vi "Read id.vi"(8 "error in (no error)":errorcluster, 11 "IDable in":refnum<class "IDable.lvclass">) -> (0 "error out":errorcluster, 2 "id":string, 3 "IDable out":refnum<class "IDable.lvclass">)   [LabVIEW 2017, in "IDable.lvclass"]
uses:
  IDable.lvclass
  IDable.lvclass/IDable.ctl
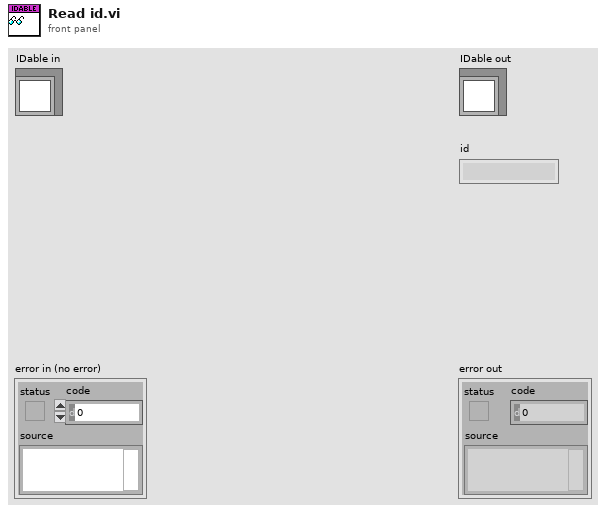
[diagram p1: front panel]
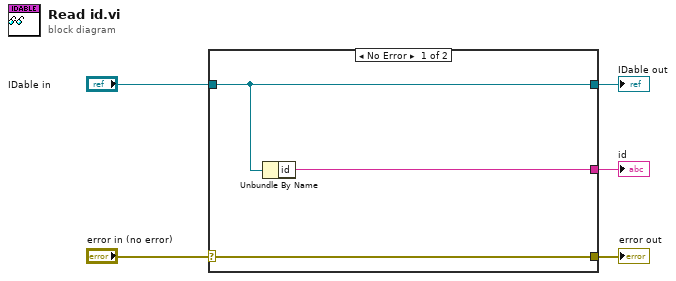
[diagram p0: block diagram]
diagram:
  n1 = case shown="No Error" "error in (no error)" {
    selector: "error in (no error)" -> [w8 w9]
    tunnel: [w8 w9] -> w4
    tunnel: [w7 w10] -> w2
    tunnel: "IDable in" -> [w7 w10]
    tunnel: [w6 _] -> w1
    frame No Error {
      n2 = Unbundle By Name(w7) -> ("id"=w6:string)
    }
    frame Error {
    }
  }
  "error out" <- w4
  "IDable out" <- w2
  "id" <- w1
